vi "read_channels_VISA.vi"(5 "postDAQ  wait ms":u32=12, 7 "preDAQ  wait ms":u32=25, 8 "error in":T1, 11 "VISA-in":refnum<visa-resource-name>="GPIB0::27::INSTR") -> (0 "error out":T1, 2 "data":dbl[](array[numeric]), 3 "VISA-out":refnum<visa-resource-name>)   [LabVIEW 2024]
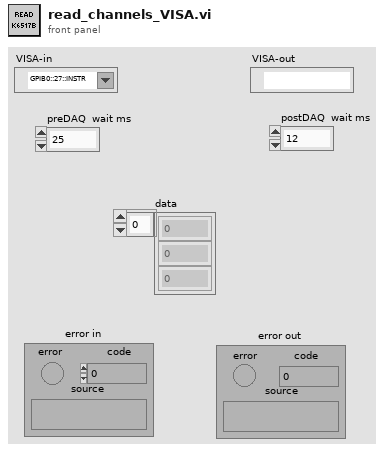
[diagram p1: front panel]
types:
  T1 = cluster{"error":bool, "code":i32, "source":string}
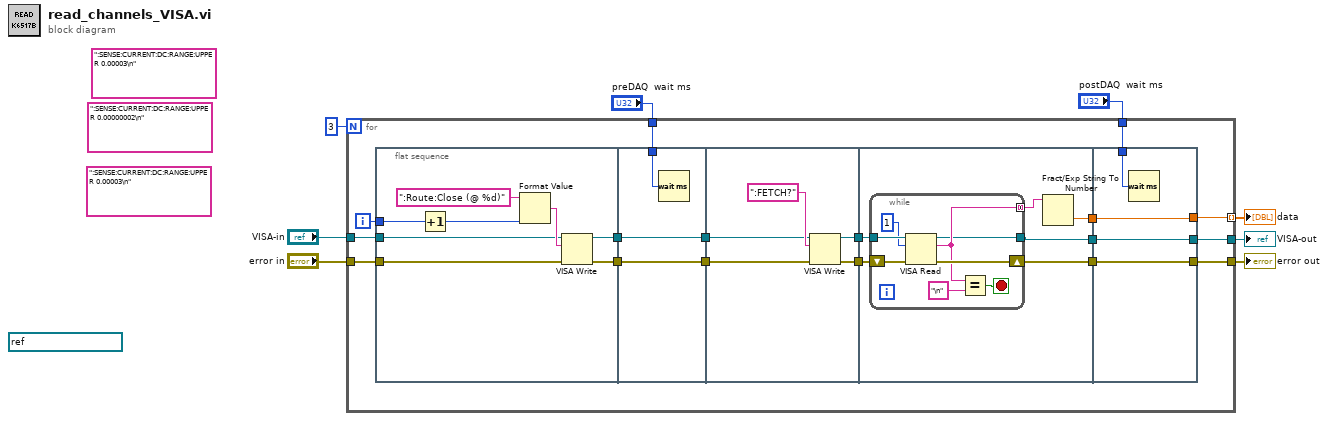
[diagram p0: block diagram]
diagram:
  (unwired) ":SENSE:CURRENT:DC:RANGE:UPPER 0.00003\n"
  (unwired) ":SENSE:CURRENT:DC:RANGE:UPPER 0.00000002\n"
  (unwired) ":SENSE:CURRENT:DC:RANGE:UPPER 0.00003\n"
  (unwired) refnum<visa-resource-name> "GPIB0::27::INSTR" ("VISA resource name")
  n1 = for {
    N: 3 -> [_]
    tunnel: "VISA-in" -> [w18]
    tunnel: "error in" -> [w17]
    tunnel: [w16] -> w5 mode=indexing
    tunnel: [w14] -> w6
    tunnel: [w12] -> w4
    tunnel: "preDAQ  wait ms" -> [w10]
    tunnel: "postDAQ  wait ms" -> [w9]
    i -> [w11]
    n2 = flat-sequence {
      tunnel: w18 -> [w31]
      tunnel: w17 -> [w30]
      tunnel: [w29] -> w25
      tunnel: [w28] -> w24
      tunnel: w11 -> [w26]
      tunnel: [w36] -> w23
      tunnel: w25 -> [w36]
      tunnel: [w35] -> w22
      tunnel: w24 -> [w35]
      tunnel: w10 -> [w34]
      tunnel: w23 -> [w40]
      tunnel: w22 -> [w39]
      tunnel: [w38] -> w21
      tunnel: [w37] -> w20
      tunnel: w21 -> [w47]
      tunnel: w20 -> [w46]
      tunnel: [w44] -> w19
      tunnel: [w43] -> w15
      tunnel: [w42] -> w13
      tunnel: [w59] -> w16
      tunnel: w19 -> [w59]
      tunnel: [w58] -> w14
      tunnel: w15 -> [w58]
      tunnel: [w57] -> w12
      tunnel: w13 -> [w57]
      tunnel: w9 -> [w56]
      frame #0 {
        n3 = Increment(x=w26) -> (x+1=w27:i32)
        n4 = Format Value(string ("")=":Route:Close (@ %d)", value (0)=w27) -> (output string=w32:string)  [unwired: 1 in]
        n5 = VISA Write(VISA resource name=w31, write buffer=w32, error in (no error)=w30) -> (VISA resource name out=w29:refnum<visa-resource-name>, error out=w28:errorcluster)  [unwired: 1 out]
      }
      frame #1 {
        n6 = Wait (ms)(milliseconds to wait=w34) -> ()  [unwired: 1 out]
      }
      frame #2 {
        n7 = VISA Write(VISA resource name=w40, write buffer=":FETCH?", error in (no error)=w39) -> (VISA resource name out=w37:refnum<visa-resource-name>, error out=w38:errorcluster)  [unwired: 1 out]
      }
      frame #3 {
        n8 = while {
          shift-right: [w54] -> w42
          shift-left: w47 -> [w55]
          tunnel: [w52] -> w45 mode=concatenating
          tunnel: w46 -> [w53]
          tunnel: [w49] -> w43
          stop <- w50 stop-if-true
          n9 = VISA Read(VISA resource name=w53, byte count=u32 1, error in (no error)=w55) -> (VISA resource name out=w49:refnum<visa-resource-name>, read buffer=w52:string, error out=w54:errorcluster)  [unwired: 1 out]
          n10 = Equal?(x=w52, y="\n") -> (x = y?=w50:bool)
        }
        n11 = Fract/Exp String To Number(string=w45) -> (number=w44:dbl)  [unwired: 3 in, 1 out]
      }
      frame #4 {
        n12 = Wait (ms)(milliseconds to wait=w56) -> ()  [unwired: 1 out]
      }
    }
  }
  "error out" <- w4
  "data" <- w5
  "VISA-out" <- w6
